vi "Swerve Wheel.vi"(2 "Wheel":T1(ring), 4 "Inputs":dbl[](array[numeric])) -> (0 "Speed":dbl)   [LabVIEW 2018]
uses:
  <vilib>/addons/control/pid/pid.llb/PID (DBL).vi
  <vilib>/addons/control/pid/NI_PID_pid.lvlib
panel:
  in  "Inputs 3":dbl[](array[numeric])
  out "Front Right angle 2":dbl=180.0 format="%#_13g"
  out "Front Right Encoder 2":dbl=180.0 format="%#_13g"
  out "Target angle FR 2":dbl=180.0 format="%#_13g"
  out "Front left angle 2":dbl=180.0 format="%#_13g"
  out "Front Left Encoder  2":dbl=180.0 format="%#_13g"
  out "fl 2":dbl=180.0 format="%#_13g"
  out "Back Right angle  2":dbl=180.0 format="%#_13g"
  out "Back Right Encoder 2":dbl=180.0 format="%#_13g"
  out "BR 2":dbl=180.0 format="%#_13g"
  out "Back left angle 2":dbl=180.0 format="%#_13g"
  out "Back Left Encoder 2":dbl=180.0 format="%#_13g"
  out "BL 2":dbl=180.0 format="%#_13g"
  out "Speed 2":dbl
  in  "Inputs 2":dbl[](array[numeric])
  out "fl":dbl=180.0 format="%#_13g"
  out "BR":dbl=180.0 format="%#_13g"
  out "BL":dbl=180.0 format="%#_13g"
  out "Target angle FR":dbl=180.0 format="%#_13g"
  out "Front Left Encoder":dbl=180.0 format="%#_13g"
  out "Back Right Encoder":dbl=180.0 format="%#_13g"
  out "Back Left Encoder":dbl=180.0 format="%#_13g"
  out "Front Right angle":dbl=180.0 format="%#_13g"
  out "Front left angle":dbl=180.0 format="%#_13g"
  out "Back Right angle":dbl=180.0 format="%#_13g"
  out "Back left angle":dbl=180.0 format="%#_13g"
  out "Front Right Encoder":dbl=180.0 format="%#_13g"
  # "Being Processed"
  # "Output"
  # "CURRENT ANGLE vs ENCODER VALUE vs TARGET ANG;E"
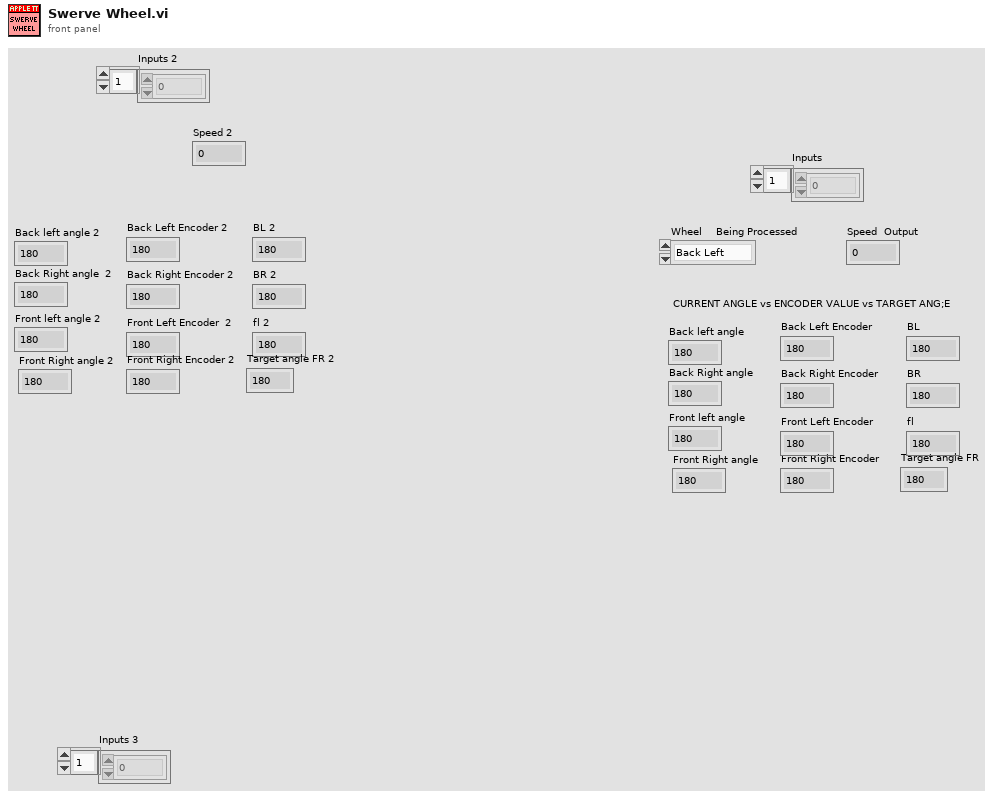
[diagram p1: front panel]
types:
  T1 = enum16{"Back Left", "Back Right", "Front Left", "Front Right"}
  T2 = enum16{"Z", "Y", "X", "Rot. Point X", "Rot. Point Y", "Width/2", "Max", "Length/2"}
  T3 = enum16{"Z Axis", "Y", "X", "Rot. Point X", "Rot. Point Y", "Width/2", "Max", "Length/2"}
  T4 = cluster{"proportional gain (Kc)":dbl, "integral time (Ti, min)":dbl, "derivative time (Td, min)":dbl}
  T5 = typedef "WPI_AnalogChannelDevRef.ctl" = cluster{"DevStatus":errorcluster, "Analog Channel":T6}
  T6 = typedef "FPGA_AIChannel.ctl" = enum8{"AI 0", "AI 1", "AI 2", "AI 3", "AI MXP 0", "AI MXP 1", "AI MXP 2", "AI MXP 3", "Invalid"}
  T7 = typedef "WPI_MotorControlDeviceRef.ctl" = cluster{"DeviceStatus":errorcluster, "Type":T8, "PWM":cluster{"PWM Channel":T9, "DeadBand":T10}, "CAN":cluster{"Device Number":u8, "SetOutput VI Ref":variant, "GetOutput VI Ref":variant, "Enable VI Ref":variant, "Disable VI Ref":variant, "Data":variant}, "Invert":bool, "DIO PWM":cluster{"PWM \"Enable\" Channel":T9, "DIOChannel":T11, "PWM Rate":dbl}}
  T8 = typedef "WPI_MotorControlType.ctl" = enum16{"PWM", "CAN", "DIO PWM"}
  T9 = typedef "FPGA_DIOPWMChannel.ctl" = enum8{"PWM 0", "PWM 1", "PWM 2", "PWM 3", "PWM 4", "PWM 5", "PWM 6", "PWM 7", "PWM 8", "PWM 9", "PWM MXP 0", "PWM MXP 1", "PWM MXP 2", "PWM MXP 3", "PWM MXP 4", "PWM MXP 5", "PWM MXP 6", "PWM MXP 7", "PWM MXP 8", "PWM MXP 9", "Invalid"}
  T10 = typedef "WPI_PWMDeadband.ctl" = cluster{"Name":string, "maxPositivePwm":i32, "minPositivePwm":i32, "centerPwm":i32, "maxNegativePwm":i32, "minNegativePwm":i32, "angularRange":u16}
  T11 = typedef "FPGA_DIOChannel.ctl" = enum8{"DIO 0", "DIO 1", "DIO 2", "DIO 3", "DIO 4", "DIO 5", "DIO 6", "DIO 7", "DIO 8", "DIO 9", "DIO MXP 0", "DIO MXP 1", "DIO MXP 2", "DIO MXP 3", "DIO MXP 4", "DIO MXP 5", "DIO MXP 6", "DIO MXP 7", "DIO MXP 8", "DIO MXP 9", "DIO MXP 10", "DIO MXP 11", "DIO MXP 12", "DIO MXP 13", "DIO MXP 14", "DIO MXP 15", "SPI Port CS1", "SPI Port CS2", "SPI Port CS3", "SPI Port MISO", "SPI Port MOSI", "Invalid"}
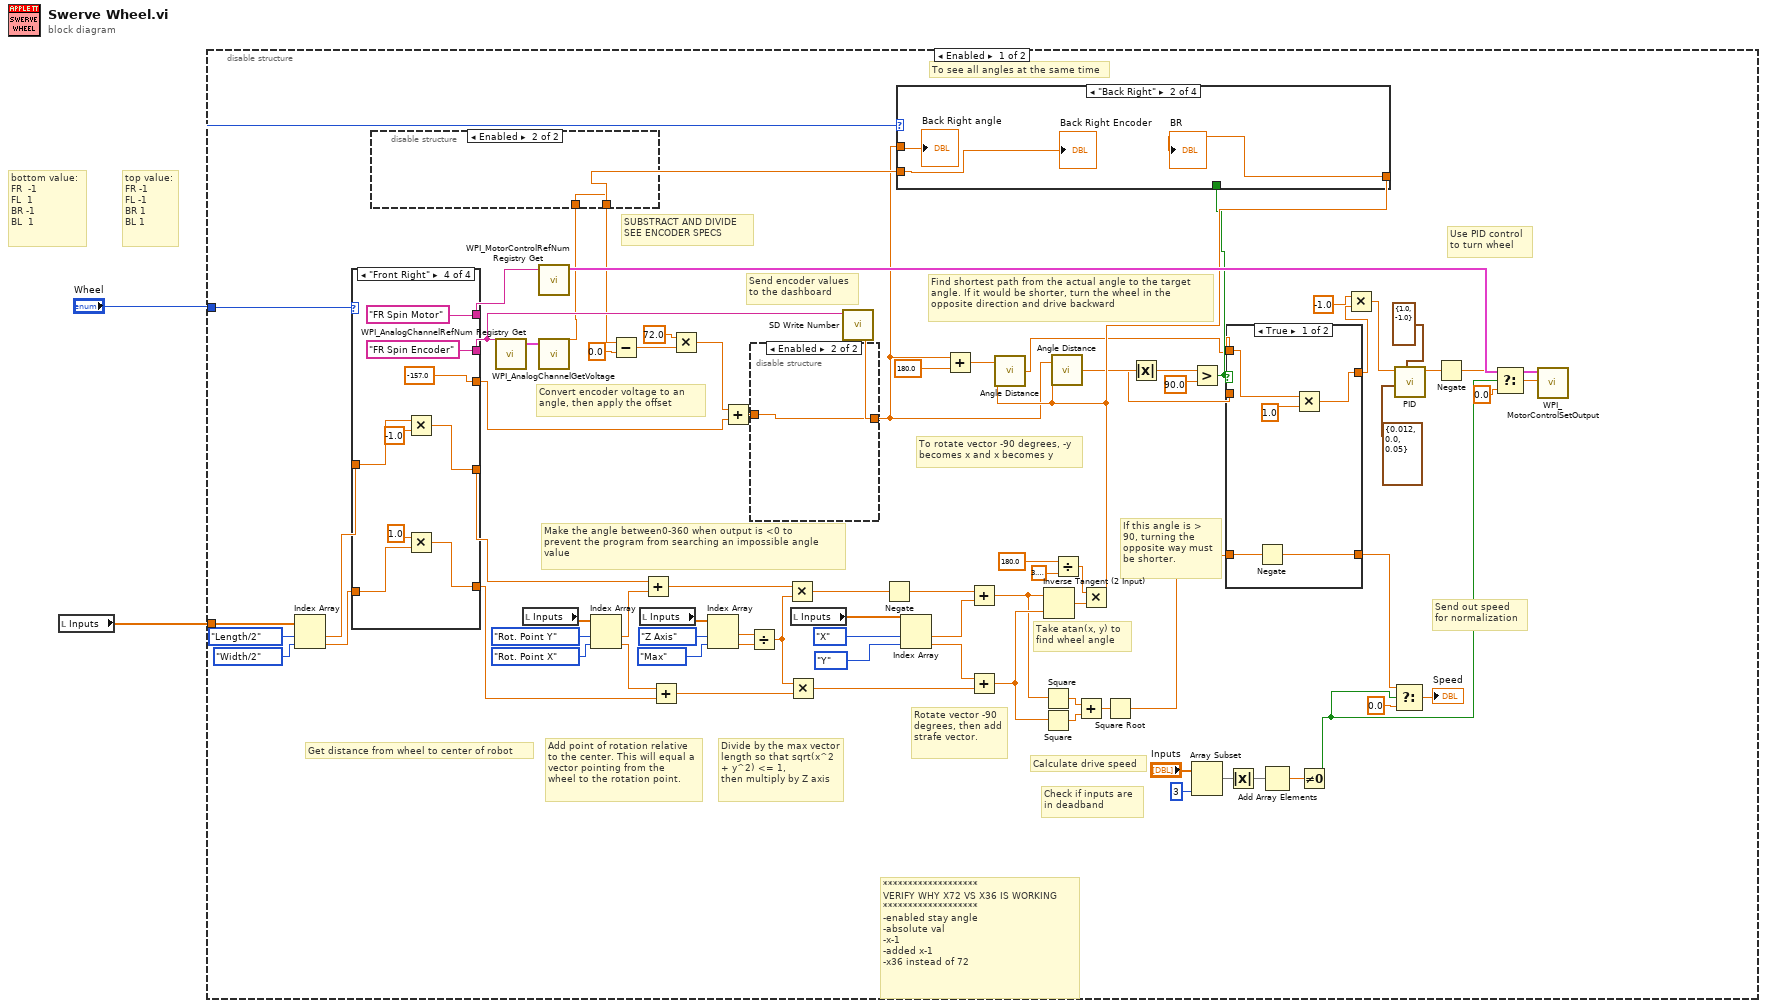
[diagram p0: block diagram]
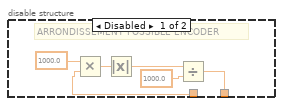
[diagram p2: hidden frame]
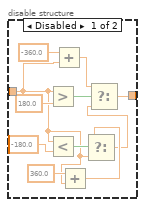
[diagram p3: hidden frame]
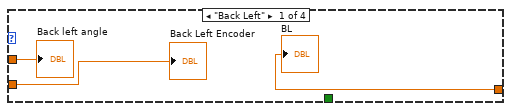
[diagram p4: hidden frame]
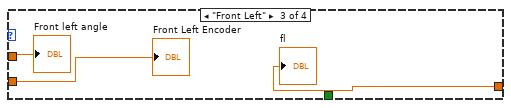
[diagram p5: hidden frame]
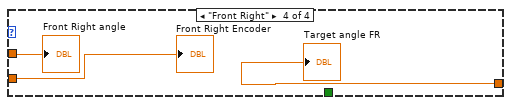
[diagram p6: hidden frame]
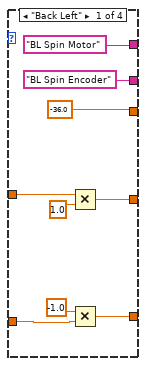
[diagram p8: hidden frame]
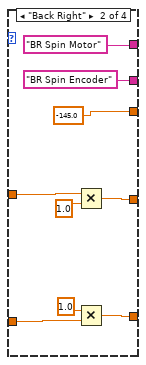
[diagram p9: hidden frame]
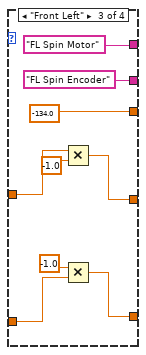
[diagram p10: hidden frame]
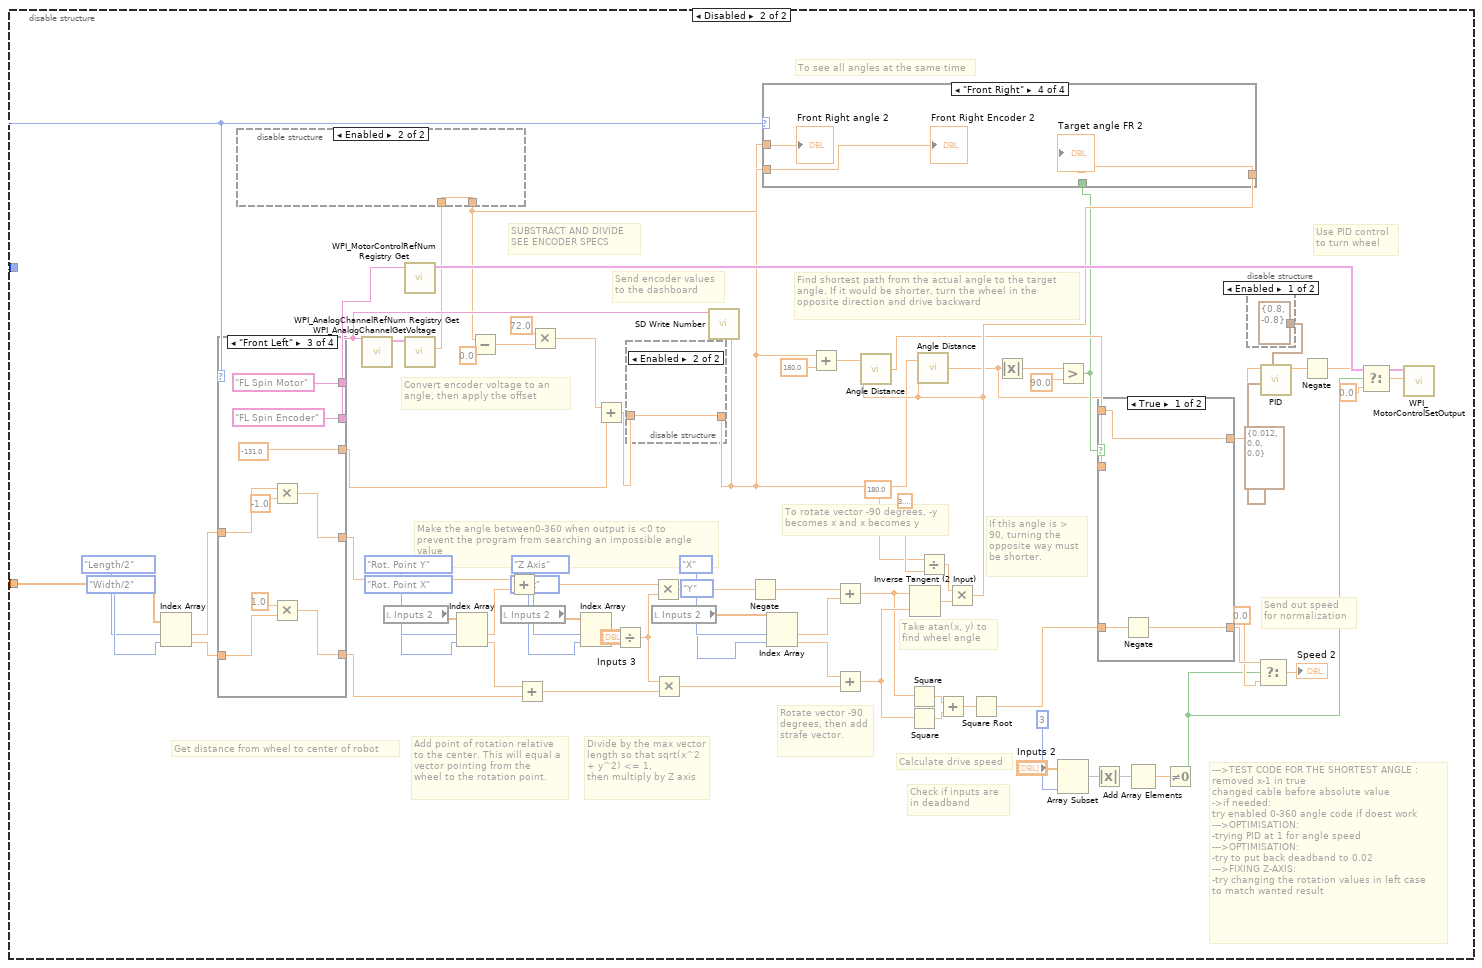
[diagram p11: hidden frame]
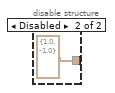
[diagram p12: hidden frame]
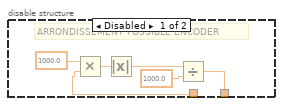
[diagram p13: hidden frame]
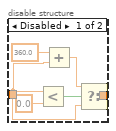
[diagram p14: hidden frame]
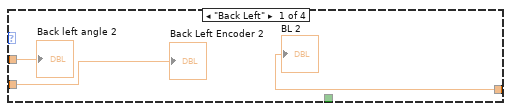
[diagram p15: hidden frame]
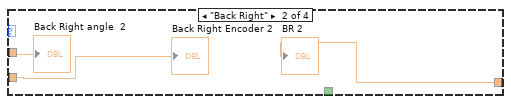
[diagram p16: hidden frame]
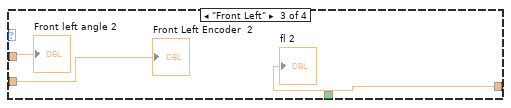
[diagram p17: hidden frame]
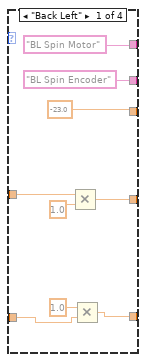
[diagram p19: hidden frame]
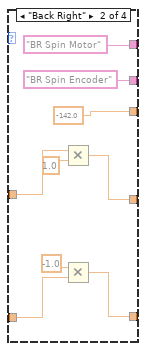
[diagram p20: hidden frame]
diagram:
  # "top value:\nFR -1 \nFL -1\nBR 1\nBL 1"
  # "bottom value:\nFR  -1 \nFL  1\nBR -1\nBL  1"
  n1 = local read "Inputs"() -> (w2:dbl[])
  n2 = disable-structure shown="Enabled" {
    disable-tunnel: "Wheel" -> [w11 w156]
    disable-tunnel: w2 -> [w10 w155]
    frame Enabled {
      # "*******************\nVERIFY WHY X72 VS X36 IS WORKING\n*******************\n-enabled stay angle\n-absolute val\n-x-1\n-added x-1\n-x36 instead of 72"
      # "SUBSTRACT AND DIVIDE\nSEE ENCODER SPECS"
      # "Make the angle between0-360 when output is <0 to\nprevent the program from searching an impossible angle\nvalue"
      # "To see all angles at the same time"
      # "Send encoder values \nto the dashboard"
      # "To rotate vector -90 degrees, -y becomes x and x becomes y"
      # "Divide by the max vector length so that sqrt(x^2 + y^2) <= 1,\nthen multiply by Z axis"
      # "Add point of rotation relative to the center. This will equal a vector pointing from the\nwheel to the rotation point."
      # "Send out speed\nfor normalization"
      # "Check if inputs are\nin deadband"
      # "Convert encoder voltage to an angle, then apply the offset"
      # "If this angle is > 90, turning the opposite way must be shorter."
      # "Use PID control\nto turn wheel"
      # "Find shortest path from the actual angle to the target angle. If it would be shorter, turn the wheel in the opposite direction and drive backward"
      # "Take atan(x, y) to find wheel angle"
      # "Calculate drive speed"
      # "Rotate vector -90 degrees, then add strafe vector."
      # "Get distance from wheel to center of robot"
      n3 = Index Array(array=w10, index #1=T2."Length/2", index #2=T2."Width/2") -> (element #1=w26:dbl, element #2=w25:dbl)
      n4 = case shown="\"Front Right\"" w11 {
        tunnel: ["BL Spin Encoder" "BR Spin Encoder" "FL Spin Encoder" "FR Spin Encoder"] -> w54
        tunnel: ["BL Spin Motor" "BR Spin Motor" "FL Spin Motor" "FR Spin Motor"] -> w68
        tunnel: [-36.0 ("y") -145.0 ("y") -134.0 ("y") -157.0 ("y")] -> w7
        tunnel: w26 -> [w124 w133 w142 w151]
        tunnel: w25 -> [w122 w131 w140 w149]
        tunnel: [w121 w130 w139 w148] -> w51
        tunnel: [w120 w129 w138 w147] -> w47
        frame "Back Left" {
          n5 = Multiply(x=w124, y=1.0) -> (x*y=w121:dbl)
          n6 = Multiply(x=-1.0 ("y"), y=w122) -> (x*y=w120:dbl)
        }
        frame "Back Right" {
          n7 = Multiply(x=w133, y=1.0) -> (x*y=w130:dbl)
          n8 = Multiply(x=1.0 ("y"), y=w131) -> (x*y=w129:dbl)
        }
        frame "Front Left" {
          n9 = Multiply(x=w142, y=-1.0) -> (x*y=w139:dbl)
          n10 = Multiply(x=-1.0 ("y"), y=w140) -> (x*y=w138:dbl)
        }
        frame "Front Right" {
          n11 = Multiply(x=w151, y=-1.0) -> (x*y=w148:dbl)
          n12 = Multiply(x=1.0 ("y"), y=w149) -> (x*y=w147:dbl)
        }
      }
      n13 = call <vilib>:"WPI_AnalogChannelRefNum Registry Get.vi"("refnum name"=w54) -> ("AIDeviceRef"=w64:T5)  [unwired: 9 in, 1 out]
      n14 = local read "Inputs"() -> (w49:dbl[])
      n15 = call <vilib>:"WPI_MotorControlRefNum Registry Get.vi"("refnum name"=w68) -> ("MotorControlDevRef"=w78:T7)  [unwired: 9 in, 1 out]
      n16 = call <vilib>:"WPI_AnalogChannelGetVoltage.vi"("AIDeviceRef"=w64) -> ("Voltage"=w12:dbl)  [unwired: 8 in, 2 out]
      n17 = disable-structure shown="Enabled" {
        disable-tunnel: [w84 w87] -> w18
        disable-tunnel: w12 -> [w82 w87]
        frame Disabled {
          # "ARRONDISSEMENT POSSIBLE ENCODER"
          n18 = Multiply(x=1000.0 ("y"), y=w82) -> (x*y=w85:dbl)
          n19 = Absolute Value(x=w85) -> (abs(x)=w86:dbl)
          n20 = Divide(x=w86, y=1000.0) -> (x/y=w84:dbl)
        }
        frame Enabled {
        }
      }
      n21 = Index Array(array=w49, index #1=T2."Rot. Point Y", index #2=T2."Rot. Point X") -> (element #1=w45:dbl, element #2=w46:dbl)
      n22 = Subtract(x=w18, y=0.0) -> (x-y=w63:dbl)
      n23 = local read "Inputs"() -> (w43:dbl[])
      n24 = Add(x=w51, y=w45) -> (x+y=w22:dbl)
      n25 = Add(x=w46, y=w47) -> (x+y=w39:dbl)
      n26 = Multiply(x=72.0 ("y"), y=w63) -> (x*y=w20:dbl)
      n27 = Index Array(array=w43, index #1=T3."Z Axis", index #2=T2."Max") -> (element #1=w40:dbl, element #2=w41:dbl)
      n28 = Add(x=w20, y=w7) -> (x+y=w15:dbl)
      n29 = Divide(x=w40, y=w41) -> (x/y=w38:dbl)
      n30 = disable-structure shown="Enabled" {
        disable-tunnel: [w96 w99] -> w16
        disable-tunnel: w15 -> [w89 w99]
        frame Disabled {
          n31 = Greater?(x=w89, y=180.0) -> (0:w97:bool)
          n32 = Less?(x=w89, y=-180.0) -> (x < y?=w92:bool)
          n33 = Add(x=-360.0 ("y"), y=w89) -> (x+y=w95:dbl)
          n34 = Add(x=360.0 ("y"), y=w89) -> (x+y=w90:dbl)
          n35 = Select(t=w90, s=w92, f=w89) -> (s? t:f=w88:dbl)
          n36 = Select(t=w95, s=w97, f=w88) -> (s? t:f=w96:dbl)
        }
        frame Enabled {
        }
      }
      n37 = Multiply(x=w22, y=w38) -> (x*y=w24:dbl)
      n38 = Multiply(x=w38, y=w39) -> (x*y=w33:dbl)
      n39 = local read "Inputs"() -> (w36:dbl[])
      n40 = call <vilib>:"SD Write Number.vi"("Numeric"=w16, "Name"=w54) -> ()  [unwired: 8 in, 2 out]
      n41 = Negate(x=w24) -> (-x=w23:dbl)
      n42 = Index Array(array=w36, index #1=T2."X", index #2=T2."Y") -> (element #1=w31:dbl, element #2=w32:dbl)
      n43 = Add(x=w16, y=180.0 ("f")) -> (x+y=w17:dbl)
      n44 = Add(x=w23, y=w31) -> (x+y=w29:dbl)
      n45 = Add(x=w32, y=w33) -> (x+y=w30:dbl)
      n46 = Square(x=w29) -> (x^2=w34:dbl)
      n47 = Square(x=w30) -> (x^2=w75:dbl)
      n48 = Inverse Tangent (2 Input)(1:w30, 2:w29) -> (0:w76:dbl)
      n49 = Divide(x=180.0 ("y"), y=3.141592653589793) -> (x/y=w73:dbl)
      n50 = Add(x=w34, y=w75) -> (x+y=w74:dbl)
      n51 = Multiply(x=w73, y=w76) -> (x*y=w19:dbl)
      n52 = call "Angle Distance.vi"("target angle"=w19, "current angle"=w17) -> ("distance"=w6:dbl)
      n53 = call "Angle Distance.vi"("target angle"=w19, "current angle"=w16) -> ("distance"=w9:dbl)
      n54 = Square Root(x=w74) -> (sqrt(x)=w69:dbl)
      n55 = Absolute Value(x=w9) -> (abs(x)=w8:dbl)
      n56 = Greater?(x=w8, y=90.0) -> (0:w13:bool)
      n57 = case shown="\"Back Right\"" w11 {
        tunnel: w16 -> [w102 w105 w108 w111]
        tunnel: w18 -> [w101 w104 w107 w110]
        tunnel: w19 -> [w100 w103 w106 w109]
        tunnel: w13 -> [_ _ _ _]
        frame "Back Left" {
          "Back left angle" <- w102
          "Back Left Encoder" <- w101
          "BL" <- w100
        }
        frame "Back Right" {
          "Back Right angle" <- w105
          "Back Right Encoder" <- w104
          "BR" <- w103
        }
        frame "Front Left" {
          "Front left angle" <- w108
          "Front Left Encoder" <- w107
          "fl" <- w106
        }
        frame "Front Right" {
          "Front Right angle" <- w111
          "Front Right Encoder" <- w110
          "Target angle FR" <- w109
        }
      }
      n58 = Array Subset(array="Inputs", length=3) -> (w59:dbl[])  [unwired: 1 in]
      n59 = case shown="True" w13 {
        tunnel: w6 -> [w113 _]
        tunnel: [w115 w118] -> w58
        tunnel: w69 -> [w116 w118]
        tunnel: [w112 w117] -> w3
        tunnel: w8 -> [_ w117]
        frame True {
          n60 = Negate(x=w116) -> (-x=w115:dbl)
          n61 = Multiply(x=w113, y=1.0) -> (x*y=w112:dbl)
        }
        frame False {
        }
      }
      n62 = Absolute Value(x=w59) -> (abs(x)=w52:dbl[])
      n63 = Add Array Elements(numeric array=w52) -> (sum=w77:dbl)
      n64 = Not Equal To 0?(x=w77) -> (x != 0?=w55:bool)
      n65 = Multiply(x=-1.0 ("output low"), y=w3) -> (x*y=w4:dbl)
      n66 = Select(t=w58, s=w55, f=0.0) -> (s? t:f=→"Speed":dbl)
      n67 = call-poly <vilib>:"PID.vi"("output range"=cluster{"output high":dbl, "output low":dbl} {"output high"=1.0, "output low"=-1.0}, "PID gains"=T4 {"proportional gain (Kc)"=0.012, "integral time (Ti, min)"=0.0, "derivative time (Td, min)"=0.05}, "setpoint"=w4) -> ("output"=w60:dbl)  [unwired: 7 in, 1 out]
      n68 = Negate(x=w60) -> (-x=w53:dbl)
      n69 = Select(t=w53, s=w55, f=0.0) -> (s? t:f=w61:dbl)
      n70 = call <vilib>:"WPI_MotorControlSetOutput.vi"("Output"=w61, "MotorControlDevRef"=w78) -> ()  [unwired: 7 in, 3 out]
    }
    frame Disabled {
      # "--->TEST CODE FOR THE SHORTEST ANGLE :\nremoved x-1 in true\nchanged cable before absolute value\n->if needed:\ntry enabled 0-360 angle code if doest work\n--->OPTIMISATION:\n-trying PID at 1 for angle speed\n--->OPTIMISATION:\n-try to put back deadband to 0.02\n--->FIXING Z-AXIS:\n-try changing the rotation values in left case\nto match wanted result"
      # "SUBSTRACT AND DIVIDE\nSEE ENCODER SPECS"
      # "Make the angle between0-360 when output is <0 to\nprevent the program from searching an impossible angle\nvalue"
      # "To see all angles at the same time"
      # "Send encoder values \nto the dashboard"
      # "To rotate vector -90 degrees, -y becomes x and x becomes y"
      # "Divide by the max vector length so that sqrt(x^2 + y^2) <= 1,\nthen multiply by Z axis"
      # "Add point of rotation relative to the center. This will equal a vector pointing from the\nwheel to the rotation point."
      # "Send out speed\nfor normalization"
      # "Check if inputs are\nin deadband"
      # "Convert encoder voltage to an angle, then apply the offset"
      # "If this angle is > 90, turning the opposite way must be shorter."
      # "Use PID control\nto turn wheel"
      # "Find shortest path from the actual angle to the target angle. If it would be shorter, turn the wheel in the opposite direction and drive backward"
      # "Take atan(x, y) to find wheel angle"
      # "Calculate drive speed"
      # "Rotate vector -90 degrees, then add strafe vector."
      # "Get distance from wheel to center of robot"
      n71 = Index Array(array=w155, index #1=T2."Length/2", index #2=T2."Width/2") -> (element #1=w175:dbl, element #2=w174:dbl)
      n72 = case shown="\"Front Left\"" w156 {
        tunnel: ["BL Spin Encoder" "BR Spin Encoder" "FL Spin Encoder" "FR Spin Encoder"] -> w203
        tunnel: ["BL Spin Motor" "BR Spin Motor" "FL Spin Motor" "FR Spin Motor"] -> w218
        tunnel: [-23.0 ("y") -142.0 ("y") -131.0 ("y") -298.0 ("y")] -> w159
        tunnel: w175 -> [w269 w278 w287 w296]
        tunnel: w174 -> [w267 w276 w285 w294]
        tunnel: [w266 w275 w284 w293] -> w200
        tunnel: [w265 w274 w283 w292] -> w196
        frame "Back Left" {
          n73 = Multiply(x=w269, y=1.0) -> (x*y=w266:dbl)
          n74 = Multiply(x=1.0 ("y"), y=w267) -> (x*y=w265:dbl)
        }
        frame "Back Right" {
          n75 = Multiply(x=w278, y=1.0) -> (x*y=w275:dbl)
          n76 = Multiply(x=-1.0 ("y"), y=w276) -> (x*y=w274:dbl)
        }
        frame "Front Left" {
          n77 = Multiply(x=w287, y=-1.0) -> (x*y=w284:dbl)
          n78 = Multiply(x=1.0 ("y"), y=w285) -> (x*y=w283:dbl)
        }
        frame "Front Right" {
          n79 = Multiply(x=w296, y=-1.0) -> (x*y=w293:dbl)
          n80 = Multiply(x=-1.0 ("y"), y=w294) -> (x*y=w292:dbl)
        }
      }
      n81 = call <vilib>:"WPI_AnalogChannelRefNum Registry Get.vi"("refnum name"=w203) -> ("AIDeviceRef"=w213:T5)  [unwired: 9 in, 1 out]
      n82 = local read "Inputs 2"() -> (w198:dbl[])
      n83 = call <vilib>:"WPI_MotorControlRefNum Registry Get.vi"("refnum name"=w218) -> ("MotorControlDevRef"=w228:T7)  [unwired: 9 in, 1 out]
      n84 = call <vilib>:"WPI_AnalogChannelGetVoltage.vi"("AIDeviceRef"=w213) -> ("Voltage"=w160:dbl)  [unwired: 8 in, 2 out]
      n85 = disable-structure shown="Enabled" {
        disable-tunnel: [w236 w239] -> w167
        disable-tunnel: w160 -> [w234 w239]
        frame Disabled {
          # "ARRONDISSEMENT POSSIBLE ENCODER"
          n86 = Multiply(x=1000.0 ("y"), y=w234) -> (x*y=w237:dbl)
          n87 = Absolute Value(x=w237) -> (abs(x)=w238:dbl)
          n88 = Divide(x=w238, y=1000.0) -> (x/y=w236:dbl)
        }
        frame Enabled {
        }
      }
      n89 = Index Array(array=w198, index #1=T2."Rot. Point Y", index #2=T2."Rot. Point X") -> (element #1=w194:dbl, element #2=w195:dbl)
      n90 = Subtract(x=w167, y=0.0) -> (x-y=w212:dbl)
      n91 = local read "Inputs 2"() -> (w192:dbl[])
      n92 = Add(x=w200, y=w194) -> (x+y=w171:dbl)
      n93 = Add(x=w195, y=w196) -> (x+y=w188:dbl)
      n94 = Multiply(x=72.0 ("y"), y=w212) -> (x*y=w169:dbl)
      n95 = Index Array(array=w192, index #1=T3."Z Axis", index #2=T2."Max") -> (element #1=w189:dbl, element #2=w190:dbl)
      n96 = Add(x=w169, y=w159) -> (x+y=w163:dbl)
      n97 = Divide(x=w189, y=w190) -> (x/y=w187:dbl)
      n98 = disable-structure shown="Enabled" {
        disable-tunnel: [w243 w246] -> w164
        disable-tunnel: w163 -> [w242 w246]
        frame Disabled {
          n99 = Less?(x=w242, y=0.0) -> (x < y?=w244:bool)
          n100 = Add(x=360.0 ("y"), y=w242) -> (x+y=w241:dbl)
          n101 = Select(t=w241, s=w244, f=w242) -> (s? t:f=w243:dbl)
        }
        frame Enabled {
        }
      }
      n102 = local read "Inputs 2"() -> (w185:dbl[])
      n103 = Multiply(x=w171, y=w187) -> (x*y=w173:dbl)
      n104 = Multiply(x=w187, y=w188) -> (x*y=w182:dbl)
      n105 = call <vilib>:"SD Write Number.vi"("Numeric"=w164, "Name"=w203) -> ()  [unwired: 8 in, 2 out]
      n106 = Negate(x=w173) -> (-x=w172:dbl)
      n107 = Index Array(array=w185, index #1=T2."X", index #2=T2."Y") -> (element #1=w180:dbl, element #2=w181:dbl)
      n108 = Add(x=w164, y=180.0 ("f")) -> (x+y=w165:dbl)
      n109 = Add(x=w172, y=w180) -> (x+y=w178:dbl)
      n110 = Add(x=w181, y=w182) -> (x+y=w179:dbl)
      n111 = Square(x=w178) -> (x^2=w183:dbl)
      n112 = Square(x=w179) -> (x^2=w225:dbl)
      n113 = Inverse Tangent (2 Input)(1:w179, 2:w178) -> (0:w226:dbl)
      n114 = Divide(x=180.0 ("y"), y=3.141592653589793) -> (x/y=w223:dbl)
      n115 = Add(x=w183, y=w225) -> (x+y=w224:dbl)
      n116 = Multiply(x=w223, y=w226) -> (x*y=w168:dbl)
      n117 = call "Angle Distance.vi"("target angle"=w168, "current angle"=w165) -> ("distance"=w166:dbl)
      n118 = call "Angle Distance.vi"("target angle"=w168, "current angle"=w164) -> ("distance"=w157:dbl)
      n119 = Square Root(x=w224) -> (sqrt(x)=w219:dbl)
      n120 = Absolute Value(x=w157) -> (abs(x)=w158:dbl)
      n121 = Greater?(x=w158, y=90.0) -> (0:w161:bool)
      n122 = case shown="\"Front Right\"" w156 {
        tunnel: w164 -> [w249 w252 w255 w258]
        tunnel: w167 -> [w248 w251 w254 w257]
        tunnel: w168 -> [w247 w250 w253 w256]
        tunnel: w161 -> [_ _ _ _]
        frame "Back Left" {
          "Back left angle 2" <- w249
          "Back Left Encoder 2" <- w248
          "BL 2" <- w247
        }
        frame "Back Right" {
          "Back Right angle  2" <- w252
          "Back Right Encoder 2" <- w251
          "BR 2" <- w250
        }
        frame "Front Left" {
          "Front left angle 2" <- w255
          "Front Left Encoder  2" <- w254
          "fl 2" <- w253
        }
        frame "Front Right" {
          "Front Right angle 2" <- w258
          "Front Right Encoder 2" <- w257
          "Target angle FR 2" <- w256
        }
      }
      n123 = Array Subset(array="Inputs 2", length=3) -> (w208:dbl[])  [unwired: 1 in]
      n124 = Absolute Value(x=w208) -> (abs(x)=w201:dbl[])
      n125 = case shown="True" w161 {
        tunnel: w166 -> [w259 _]
        tunnel: [w260 w263] -> w207
        tunnel: w219 -> [w261 w263]
        tunnel: [w259 w262] -> w215
        tunnel: w157 -> [_ w262]
        frame True {
          n126 = Negate(x=w261) -> (-x=w260:dbl)
        }
        frame False {
        }
      }
      n127 = Add Array Elements(numeric array=w201) -> (sum=w227:dbl)
      n128 = Not Equal To 0?(x=w227) -> (x != 0?=w204:bool)
      n129 = disable-structure shown="Enabled" {
        disable-tunnel: [cluster{"output high":dbl, "output low":dbl} {"output high"=0.8, "output low"=-0.8} ("output range") cluster{"output high":dbl, "output low":dbl} {"output high"=1.0, "output low"=-1.0} ("output range")] -> w217
        frame Enabled {
        }
        frame Disabled {
        }
      }
      n130 = Select(t=w207, s=w204, f=0.0) -> (s? t:f=→"Speed 2":dbl)
      n131 = call-poly <vilib>:"PID.vi"("output range"=w217, "PID gains"=T4 {"proportional gain (Kc)"=0.012, "integral time (Ti, min)"=0.0, "derivative time (Td, min)"=0.0}, "setpoint"=w215) -> ("output"=w209:dbl)  [unwired: 7 in, 1 out]
      n132 = Negate(x=w209) -> (-x=w202:dbl)
      n133 = Select(t=w202, s=w204, f=0.0) -> (s? t:f=w210:dbl)
      n134 = call <vilib>:"WPI_MotorControlSetOutput.vi"("Output"=w210, "MotorControlDevRef"=w228) -> ()  [unwired: 7 in, 3 out]
    }
  }
